vi "20170516-lecture4-2 prof MyMenu.vi"() -> ()   [LabVIEW 2014]
panel:
  in  "stop":bool
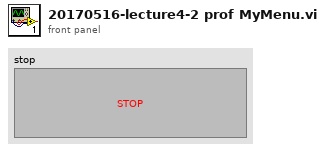
[diagram p1: front panel]
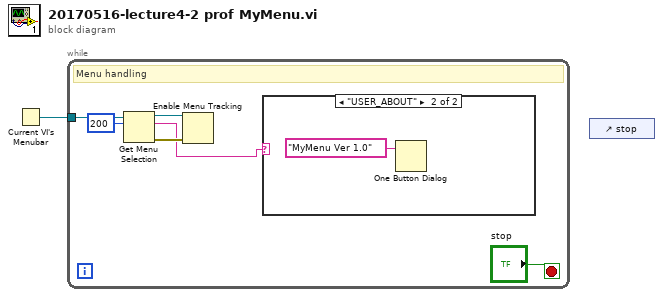
[diagram p0: block diagram]
diagram:
  n1 = Current VI's Menubar() -> (w1:refnum<k9>)
  n2 = while {
    tunnel: w1 -> [w4]
    stop <- "stop" stop-if-true
    # "Menu handling"
    n3 = Get Menu Selection(0:w4, 1:200 ("ms timeout (200)")) -> (5:w5:refnum<k9>, 6:w2:string, 8:w6:errorcluster)  [unwired: 2 in, 2 out]
    n4 = Enable Menu Tracking(2:w6, 4:w5) -> ()  [unwired: 1 in, 2 out]
    n5 = case shown="\"USER_ABOUT\"" w2 {
      frame "\u0000", Default {
      }
      frame "USER_ABOUT" {
        n6 = One Button Dialog(message="MyMenu Ver 1.0") -> ()  [unwired: 1 in, 1 out]
      }
    }
  }
  n7 = control-ref of="stop"() -> ()  [unwired: 1 out]
